vi "Create DUT Setup Sequence Step.vi"(8 "error in (no error)":errorcluster, 11 "QPA Measurement in":refnum<class "QPA Measurement.lvclass">) -> (0 "error out":errorcluster, 3 "QPA Measurement out":refnum<class "QPA Measurement.lvclass">)   [LabVIEW 2016, in "QPA Measurement.lvlib" / "QPA Measurement.lvclass"]
uses:
  QPA Measurement.lvclass
  QPA Measurement.lvclass/QPA Measurement.ctl
  Plugins/TestStand API Tools (TSAT).lvlibp/Sequence Actions/TSAT Sequence Actions.lvlib
  Plugins/TestStand API Tools (TSAT).lvlibp/Step Actions/TSAT Step Actions.lvlib
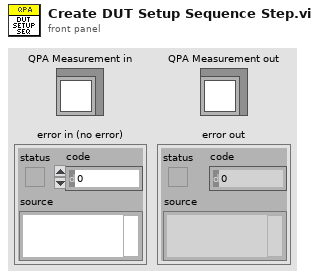
[diagram p1: front panel]
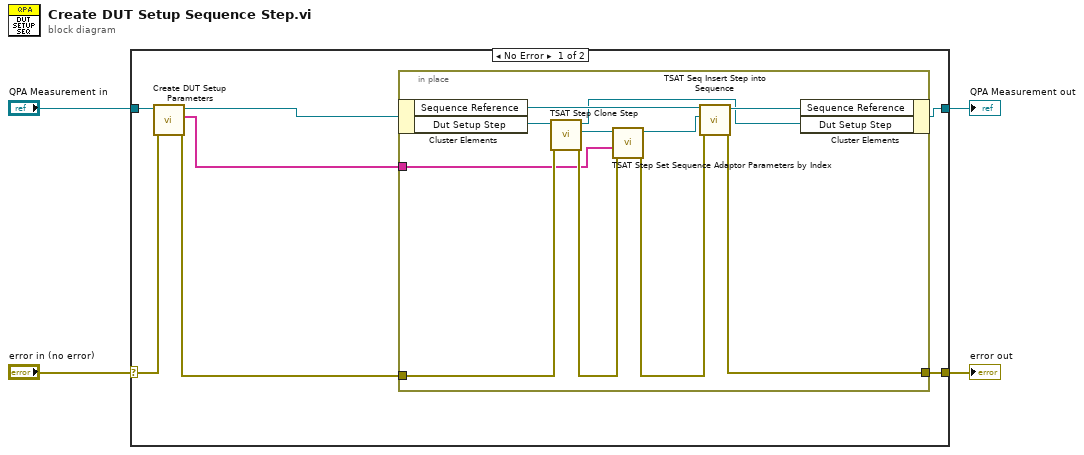
[diagram p0: block diagram]
diagram:
  n1 = case shown="No Error" "error in (no error)" {
    selector: "error in (no error)" -> [w11 w24]
    tunnel: [w5 w24] -> w3
    tunnel: [w10 w23] -> w1
    tunnel: "QPA Measurement in" -> [w8 w23]
    frame No Error {
      n2 = call "Create DUT Setup Parameters.vi"("error in (no error)"=w11, "QPA Measurement in"=w8) -> ("error out"=w9:errorcluster, "DUT Setup Parameters"=w6:string[], "QPA Measurement out"=w7:refnum<class "QPA Measurement.lvclass">)  [unwired: 7 in]
      n3 = in-place {
        in-place-border: w9 -> [w18]
        in-place-border: w6 -> [w13]
        in-place-border: [w20] -> w5
        n4 = in-place-cluster #1(w7) -> ("Sequence Reference"=w22:refnum<k7>, "Dut Setup Step"=w19:refnum<k7>)
        n5 = call "TSAT Step Clone Step.vi"("Error In"=w18, "Step In"=w19) -> ("Error Out"=w15:errorcluster, "Cloned Step"=w17:refnum<k7>, "Step Out"=w12:refnum<k7>)  [unwired: 7 in]
        n6 = call "TSAT Step Set Sequence Adaptor Parameters by Index.vi"("error in"=w15, "Parameter Array"=w13, "Step In"=w17) -> ("Error Out"=w14:errorcluster, "Step Out"=w16:refnum<k7>)  [unwired: 7 in]
        n7 = call "TSAT Seq Insert Step into Sequence.vi"("Error in"=w14, "Step to Add"=w16, "Sequence In"=w22) -> ("error out"=w20:errorcluster, "Sequence Out"=w21:refnum<k7>)  [unwired: 7 in]
        n8 = in-place-cluster #1("Sequence Reference"=w21, "Dut Setup Step"=w12) -> (w10:refnum<class "QPA Measurement.lvclass">)
      }
    }
    frame Error {
    }
  }
  "error out" <- w3
  "QPA Measurement out" <- w1
